vi "PDLM_StorePreset.vi"(8 "error in (no error)":errorcluster, 9 "PsInfo":string, 10 "PsIdx":u32, 11 "USBIdx":i32) -> (0 "error out":errorcluster, 3 "return type":i32)   [LabVIEW 2017]
uses:
  PDLM_DllPath_global.vi
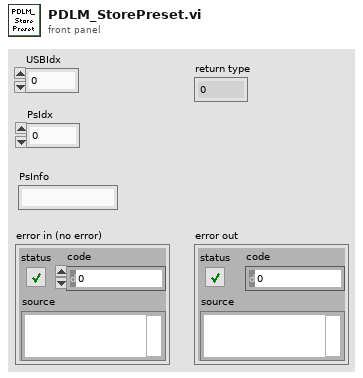
[diagram p1: front panel]
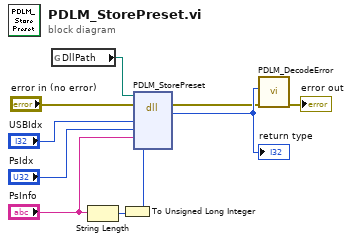
[diagram p0: block diagram]
diagram:
  n1 = global read "PDLM_DllPath_global.vi" "DllPath"() -> (w6:path)
  n2 = String Length(string="PsInfo") -> (length=w2:i32)
  n3 = To Unsigned Long Integer(number=w2) -> (unsigned 32bit integer=w1:u32)
  n4 = dll-call lib="M:/_dev/progs/LabVIEW/_lib/PQ/Taiko/pdlm_lib.dll" fn="PDLM_StorePreset"(path in=w6, error in="error in (no error)", "USBIdx"="USBIdx", "PsIdx"="PsIdx", "PsInfo"="PsInfo", "size"=w1) -> (error out=w8:errorcluster, "return type"=w9:i32)  [unwired: 5 in, 1 out]
  "return type" <- w9
  n5 = call "PDLM_DecodeError.vi"("error in (no error)"=w8, "code"=w9) -> ("error out"=→"error out":errorcluster)  [unwired: 7 in, 2 out]
